vi "BytetoBMP.vi"() -> ()   [LabVIEW 2022 SP3]
panel:
  in  "Ring":u16(ring) items=["midband", "slope", "intercept"]
  in  "pixels in y":i32=240
  in  "pixels in x":i32=256
  in  "Save to BMP?":bool
  out "data":u8[][](graph)
  out "bmp orientation":dbl[][](graph)
  # "Image assumed to be 240 X 256 which is the format for prostate parameter images."
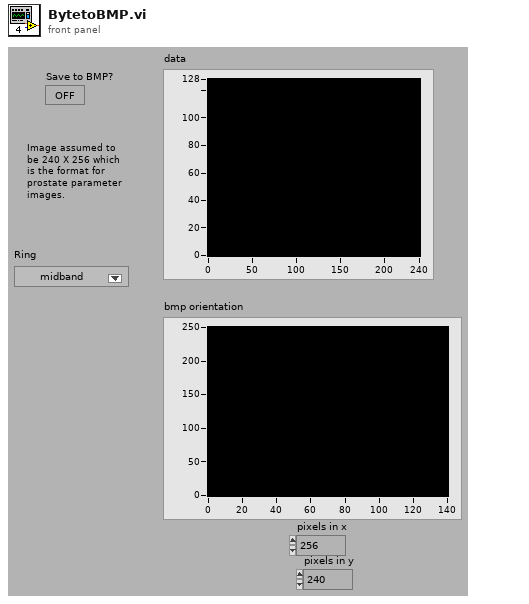
[diagram p1: front panel]
types:
  T1 = cluster{"mb max":dbl, "mb min":dbl, "slope max":dbl, "slope min":dbl, "int max":dbl, "int min":dbl}
  T2 = typedef "imagedata.ctl" = cluster{"image type":i32, "image depth":i32, "image":u8[], "mask":u8[], "colors":u32[], "Rectangle":cluster{"left":i16, "top":i16, "right":i16, "bottom":i16}}
  T3 = enum32{"existing file", "new file", "new or existing file", "existing dir", "new dir", "new or existing dir", "existing file (use LLBs)", "new file (use LLBs)", "new or existing file (use LLBs)", "new or existing file or directory (use LLBs)"}
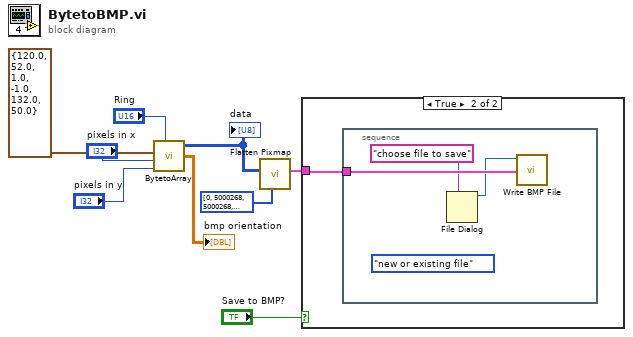
[diagram p0: block diagram]
diagram:
  n1 = call "BytetoArray.vi"("Ring"="Ring", "Range Params"=T1 {"mb max"=120.0, "mb min"=52.0, "slope max"=1.0, "slope min"=-1.0, "int max"=132.0, "int min"=50.0}, "pixels in x"="pixels in x", "pixels in y"="pixels in y") -> ("Raw data"=w7:u8[][], "Scaled data"=→"bmp orientation":dbl[][])  [unwired: 2 in, 1 out]
  "data" <- w7
  n2 = call <vilib>:"Flatten Pixmap.vi"("colors"=u32[] [0, 5000268, 5000268, 5066061, 5131854, 5131854, 5197647, 5263440, 5263440, 5329233, 5395026, 5460819, 5460819, 5526612, 5592405, 5592405, 5658198, 5723991, 5723991, 5789784, 5855577, 5921370, 5921370, 5987163, 6052956, 6052956, 6118749, 6184542, 6250335, 6250335, 6316128, 6381921, 6381921, 6447714, 6513507, 6513507, 6579300, 6645093, 6710886, 6710886, 6776679, 6842472, 6842472, 6908265, 6974058, 7039851, 7039851, 7105644, 7171437, 7171437, 7237230, 7303023, 7303023, 7368816, 7434609, 7500402, 7500402, 7566195, 7631988, 7631988, 7697781, 7763574, 7763574, 7829367, 7895160, 7960953, 7960953, 8026746, 8092539, 8092539, 8158332, 8224125, 8289918, 8289918, 8355711, 8421504, 8421504, 8487297, 8553090, 8553090, 8618883, 8684676, 8750469, 8750469, 8816262, 8882055, 8882055, 8947848, 9013641, 9079434, 9079434, 9145227, 9211020, 9211020, 9276813, 9342606, 9342606, 9408399, 9474192, 9539985, 9539985, 9605778, 9671571, 9671571, 9737364, 9803157, 9803157, 9868950, 9934743, 10000536, 10000536, 10066329, 10132122, 10132122, 10197915, 10263708, 10329501, 10329501, 10395294, 10461087, 10461087, 10526880, 10592673, 10592673, 10658466, 10724259, 10790052, 10790052, 10855845, 10921638, 10921638, 10987431, 11053224, 11119017, 11119017, 11184810, 11250603, 11250603, 11316396, 11382189, 11382189, 11447982, 11513775, 11579568, 11579568, 11645361, 11711154, 11711154, 11776947, 11842740, 11908533, 11908533, 11974326, 12040119, 12040119, 12105912, 12171705, 12171705, 12237498, 12303291, 12369084, 12369084, 12434877, 12500670, 12500670, 12566463, 12632256, 12632256, 12698049, 12763842, 12829635, 12829635, 12895428, 12961221, 12961221, 13027014, 13092807, 13158600, 13158600, 13224393, 13290186, 13290186, 13355979, 13421772, 13421772, 13487565, 13553358, 13619151, 13619151, 13684944, 13750737, 13750737, 13816530, 13882323, 13948116, 13948116, 14013909, 14079702, 14079702, 14145495, 14211288, 14211288, 14277081, 14342874, 14408667, 14408667, 14474460, 14540253, 14540253, 14606046, 14671839, 14671839, 14737632, 14803425, 14869218, 14869218, 14935011, 15000804, 15000804, 15066597, 15132390, 15198183, 15198183, 15263976, 15329769, 15329769, 15395562, 15461355, 15461355, 15527148, 15592941, 15658734, 15658734, 15724527, 15790320, 15790320, 15856113, 15921906, 15987699, 15987699, 16053492, 16119285, 16119285, 16185078, 16250871, 16250871, 16316664, 16382457, 16448250, 16448250, 16514043, 16579836, 16579836, 16645629, 16711422, 16711680] ("Array 3"), "8-bit pixmap"=w7) -> ("image data"=w9:T2)  [unwired: 4 in, 5 out]
  n3 = case shown="True" "Save to BMP?" {
    tunnel: w9 -> [_ w10]
    frame False {
    }
    frame True {
      n4 = stacked-sequence {
        tunnel: w10 -> [w13]
        frame #0 {
          (unwired) T3."new or existing file" ("select mode (2)")
          n5 = File Dialog(7:"choose file to save" ("prompt")) -> (3:w12:path)  [unwired: 1 in, 8 out]
          n6 = call <vilib>:"Write BMP File.vi"("image data"=w13, "path to BMP file"=w12) -> ()  [unwired: 2 in, 8 out]
        }
      }
    }
  }
